vi "Push Backup to DB.vi"(7 "Backup lines at a time":i32=1000, 9 "timestamp string":string, 10 "Path to backup file":path, 11 "Data.PG":refnum<class "Data.PGSQL.lvclass">) -> ()   [LabVIEW 2013, in "Data.PGSQL.lvclass"]
uses:
  Data.PGSQL.lvclass
  Data.PGSQL.lvclass/Data.PGSQL.ctl
  PostgreSQL Library/Result/PQ Result.lvclass/PQ Result.ctl
  PostgreSQL Library/Connection/Execute Command (No results).vi
  PostgreSQL Library/Result/Clear.vi
  PostgreSQL Library/Connection/Execute Command (Result).vi
  PostgreSQL Library/Connection/Execute (Return first result with rows).vi
  PostgreSQL Library/Connection/Single Command with parameters.vi
  PostgreSQL Library/Connection/PQ Connection.lvclass
panel:
  out "Success?":bool
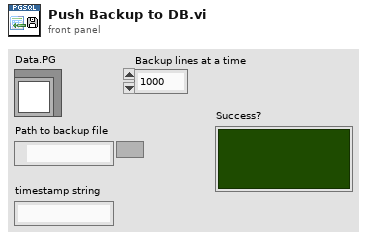
[diagram p1: front panel]
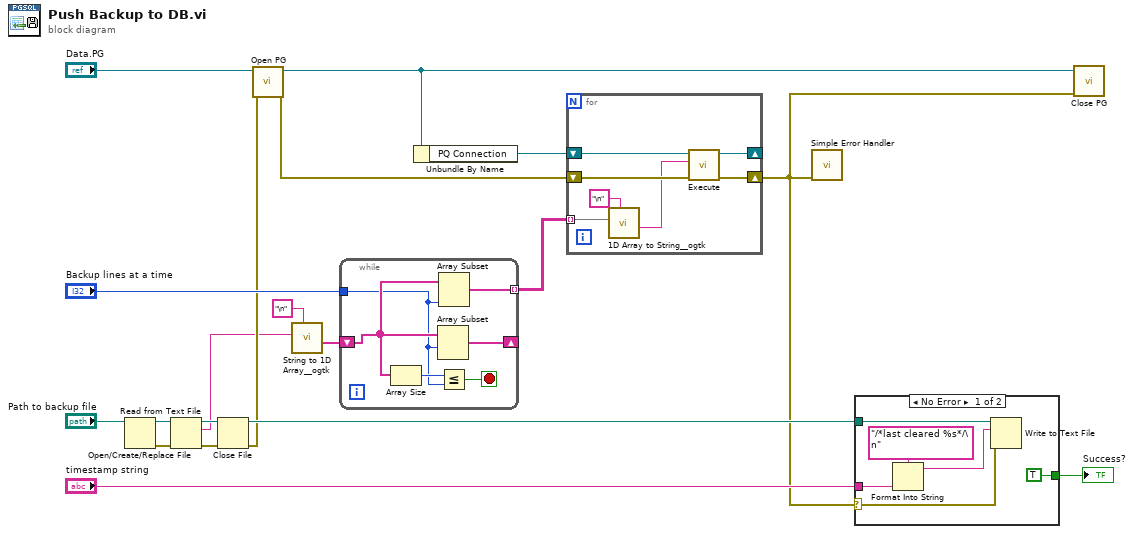
[diagram p0: block diagram]
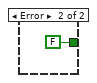
[diagram p2: hidden frame]
diagram:
  n1 = Open/Create/Replace File(file path (use dialog)="Path to backup file") -> (refnum out=w18:refnum<file>, error out=w19:errorcluster)  [unwired: 5 in, 1 out]
  n2 = Read from Text File(file (use dialog)=w18, error in=w19) -> (refnum out=w11:refnum<file>, text=w3:string, error out=w10:errorcluster)  [unwired: 2 in, 1 out]
  n3 = Close File(refnum=w11, error in=w10) -> (path=w5:path, error out=w4:errorcluster)
  n4 = call-dynamic "Open PG.vi"("error in (no error)"=w4, "Data.PG in"="Data.PG") -> ("error out"=w1:errorcluster, "Data.PG out"=w14:refnum<class "Data.PGSQL.lvclass">)  [unwired: 8 in]
  n5 = call <userlib>:"String to 1D Array__ogtk.vi"("delimiter (Tab)"="\n" ("delimiter"), "string"=w3) -> ("Array of Strings"=w7:string[])  [unwired: 9 in]
  n6 = while {
    shift-right: [w25] -> _
    shift-left: w7 -> [w24]
    tunnel: [w21] -> w16 mode=indexing
    tunnel: "Backup lines at a time" -> [w20]
    stop <- w22 stop-if-true
    n7 = Array Size(array=w24) -> (size(s)=w23:i32)
    n8 = Array Subset(array=w24, index=w20) -> (w25:string[])  [unwired: 1 in]
    n9 = Array Subset(array=w24, length=w20) -> (w21:string[])  [unwired: 1 in]
    n10 = Less Or Equal?(x=w23, y=w20) -> (x <= y?=w22:bool)
  }
  n11 = Unbundle By Name(w14) -> ("PQ Connection"=w13:refnum<class "PQ Connection.lvclass">)
  n12 = for {
    tunnel: w16 -> [w28] mode=indexing
    shift-right: [w32] -> w2
    shift-left: w1 -> [w31]
    shift-right: [w30] -> _
    shift-left: w13 -> [w29]
    n13 = call <userlib>:"1D Array to String__ogtk.vi"("delimiter (Tab)"="\n" ("delimiter"), "Array of Strings"=w28) -> ("delimited string"=w26:string)  [unwired: 9 in]
    n14 = call-poly "Execute.vi"("error in (no error)"=w31, "SQL"=w26, "PQ Connection in"=w29) -> ("error out"=w32:errorcluster, "PQ Connection out"=w30:refnum<class "PQ Connection.lvclass">)  [unwired: 7 in]
  }
  n15 = call <vilib>:"Simple Error Handler.vi"("error in (no error)"=w2) -> ()  [unwired: 4 in, 5 out]
  n16 = case shown="No Error" w2 {
    selector: w2 -> [w33 _]
    tunnel: w5 -> [w36 _]
    tunnel: "timestamp string" -> [w37 _]
    tunnel: [TRUE FALSE] -> w9
    frame No Error {
      n17 = Format Into String(format string="/*last cleared %s*/\n", w37) -> (resulting string=w35:string)  [unwired: 2 in, 1 out]
      n18 = Write to Text File(file (use dialog)=w36, text=w35, error in=w33) -> ()  [unwired: 1 in, 3 out]
    }
    frame Error {
    }
  }
  "Success?" <- w9
  n19 = call-dynamic "Close PG.vi"("error in (no error)"=w2, "Data.PG in"=w14) -> ()  [unwired: 8 in, 2 out]
